vi "Query Plugin.vi"(6 "timeout (ms)":i32=5000, 8 "error in":errorcluster, 10 "plugin_name":string, 11 "gRPC ID in":T14) -> (0 "error out":errorcluster, 2 "plugin_info":T1, 3 "gRPC ID out":T14)   [LabVIEW 2021, in "CIFManagerClientWrapper.lvlib"]
uses:
  CIFManagerClientWrapper.lvlib
  <vilib>/gRPC/LabVIEW gRPC Library/Shared/grpcId.ctl
  CIF_Manager_client/RPC Messages/cif_manager_PluginInfo.ctl
  CIF_Manager_client/RPC Messages/cif_common_ShortVersion.ctl
  CIF_Manager_client/RPC Messages/cif_management_common_PluginStatusData.ctl
  CIF_Manager_client/RPC Messages/cif_management_common_PluginStatusData_PluginState.ctl
  CIF_Manager_client/RPC Messages/cif_management_common_TimingStatistics.ctl
  CIF_Manager_client/RPC Messages/cif_common_TimingStats.ctl
  CIF_Manager_client/RPC Messages/cif_management_common_FifoStatistics.ctl
  CIF_Manager_client/RPC Messages/cif_management_common_Error.ctl
  CIF_Manager_client/RPC Messages/cif_management_common_MonitorDoubles.ctl
  CIF_Manager_client/RPC Messages/cif_management_common_MonitorU64.ctl
  CIF_Manager_client/RPC Messages/cif_management_common_MonitorI64.ctl
  CIF_Manager_client/RPC Messages/cif_management_common_LoaderInfo.ctl
  CIF_Manager_client/RPC Messages/cif_management_common_LoaderType.ctl
  CIF_Manager_client/RPC Messages/cif_manager_QueryPluginRequest.ctl
  CIF_Manager_client/CIF_Manager_client.lvlib
  <vilib>/gRPC/LabVIEW gRPC Library/grpc-lvsupport-release.lvlib
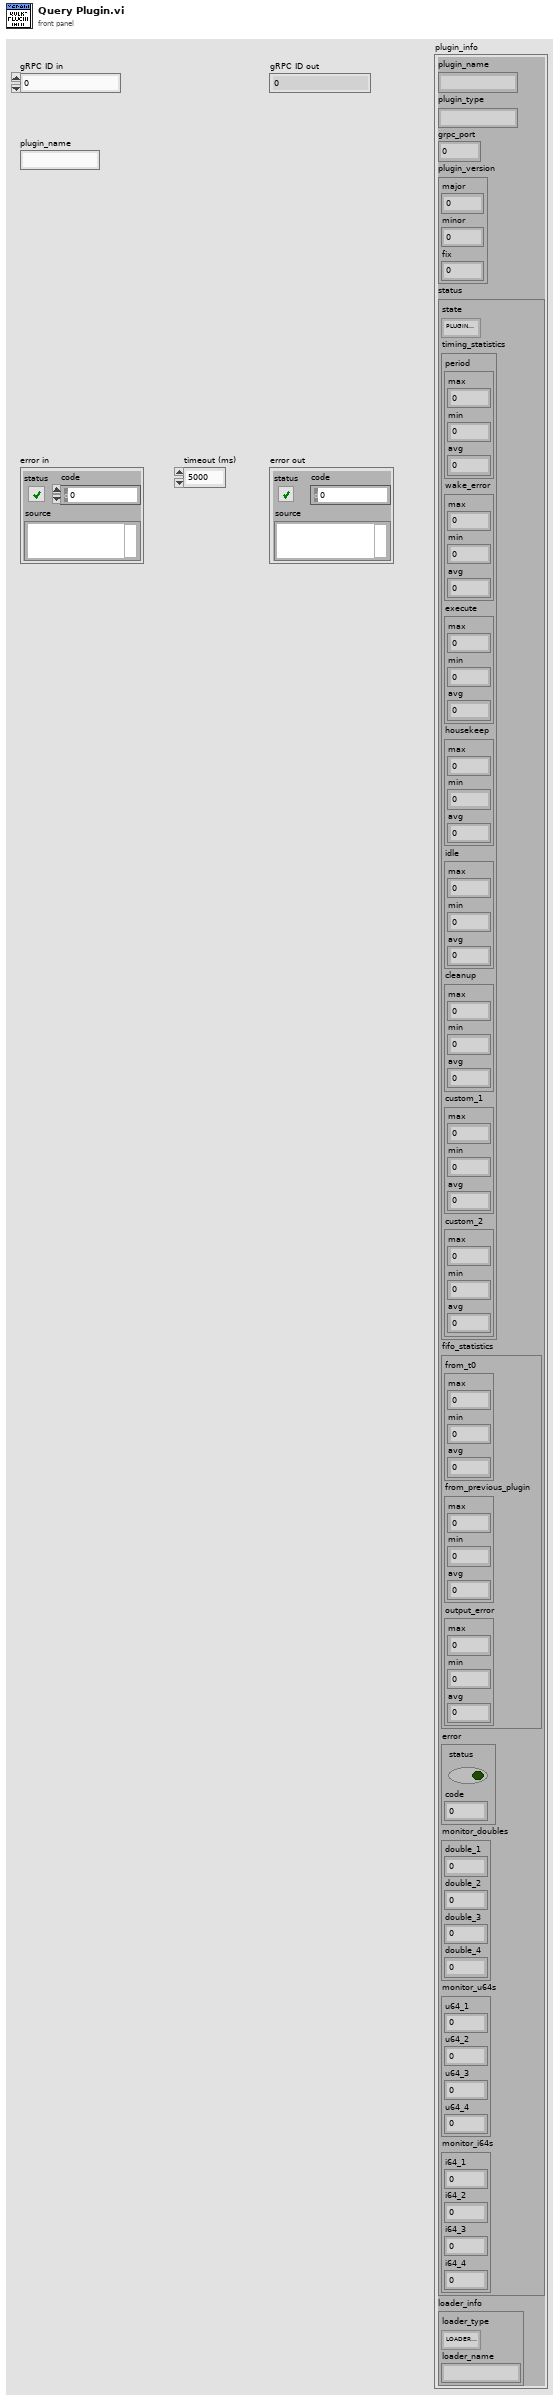
[diagram p1: front panel]
types:
  T1 = typedef "CIF_Manager_client.lvlib/cif_manager_PluginInfo.ctl" = cluster{"plugin_name":string, "plugin_type":string, "grpc_port":i32, "plugin_version":T2, "status":T3, "loader_info":T12}
  T2 = typedef "CIF_Manager_client.lvlib/cif_common_ShortVersion.ctl" = cluster{"major":u32, "minor":u32, "fix":u32}
  T3 = typedef "CIF_Manager_client.lvlib/cif_management_common_PluginStatusData.ctl" = cluster{"state":T4, "timing_statistics":T5, "fifo_statistics":T7, "error":T8, "monitor_doubles":T9, "monitor_u64s":T10, "monitor_i64s":T11}
  T4 = typedef "CIF_Manager_client.lvlib/cif_management_common_PluginStatusData_PluginState.ctl" = enum32{"PLUGINSTATE_UNKNOWN", "PLUGINSTATE_CREATING", "PLUGINSTATE_LISTENING", "PLUGINSTATE_RUNNING", "PLUGINSTATE_CLEANINGUP", "PLUGINSTATE_DESTROYING"}
  T5 = typedef "CIF_Manager_client.lvlib/cif_management_common_TimingStatistics.ctl" = cluster{"period":T6, "wake_error":T6, "execute":T6, "housekeep":T6, "idle":T6, "cleanup":T6, "custom_1":T6, "custom_2":T6}
  T6 = typedef "CIF_Manager_client.lvlib/cif_common_TimingStats.ctl" = cluster{"max":i64, "min":i64, "avg":dbl}
  T7 = typedef "CIF_Manager_client.lvlib/cif_management_common_FifoStatistics.ctl" = cluster{"from_t0":T6, "from_previous_plugin":T6, "output_error":T6}
  T8 = typedef "CIF_Manager_client.lvlib/cif_management_common_Error.ctl" = cluster{"status":bool, "code":i32}
  T9 = typedef "CIF_Manager_client.lvlib/cif_management_common_MonitorDoubles.ctl" = cluster{"double_1":dbl, "double_2":dbl, "double_3":dbl, "double_4":dbl}
  T10 = typedef "CIF_Manager_client.lvlib/cif_management_common_MonitorU64.ctl" = cluster{"u64_1":u64, "u64_2":u64, "u64_3":u64, "u64_4":u64}
  T11 = typedef "CIF_Manager_client.lvlib/cif_management_common_MonitorI64.ctl" = cluster{"i64_1":i64, "i64_2":i64, "i64_3":i64, "i64_4":i64}
  T12 = typedef "CIF_Manager_client.lvlib/cif_management_common_LoaderInfo.ctl" = cluster{"loader_type":T13, "loader_name":string}
  T13 = typedef "CIF_Manager_client.lvlib/cif_management_common_LoaderType.ctl" = enum32{"LOADERTYPE_UNKNOWN", "LOADERTYPE_LABVIEW"}
  T14 = typedef "grpc-lvsupport-release.lvlib/grpcId.ctl" = u64
  T15 = typedef "CIF_Manager_client.lvlib/cif_manager_QueryPluginRequest.ctl" = cluster{"plugin_name":string}
  T16 = typedef "CIF_Manager_client.lvlib/cif_manager_QueryPluginResponse.ctl" = cluster{"plugin_info":T1, "status":T17}
  T17 = typedef "CIF_Manager_client.lvlib/cif_common_Status.ctl" = cluster{"code":i32, "message":string}
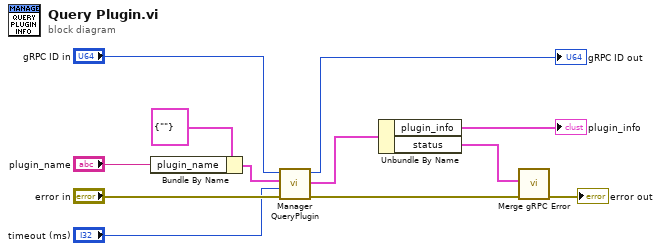
[diagram p0: block diagram]
diagram:
  n1 = Bundle By Name(cluster=T15 {"plugin_name"=""} ("Request Data"), "plugin_name"="plugin_name") -> (w3:T15)
  n2 = call "Manager QueryPlugin.vi"("error in"="error in", "timeout (ms)"="timeout (ms)", "Request Data"=w3, "gRPC ID"="gRPC ID in") -> ("error out"=w6:errorcluster, "Response Data"=w8:T16, "gRPC ID out"=→"gRPC ID out":T14)  [unwired: 5 in]
  n3 = Unbundle By Name(w8) -> ("plugin_info"=→"plugin_info":T1, "status"=w2:T17)
  n4 = call "Merge gRPC Error.vi"("error in (no error)"=w6, "gRPC Error"=w2) -> ("error out"=→"error out":errorcluster)  [unwired: 9 in]
